vi "BottomStacking.vi"(8 "Activating Button":bool, 11 "Cancel Button":bool) -> ()   [LabVIEW 2014]
uses:
  BottomStacking.ctl
  Robot Global Data.vi
  <vilib>/Rock Robotics/WPI/RobotDrive/WPI_RobotDriveGetSetRefNum.vi
  <vilib>/Rock Robotics/WPI/RobotDrive/WPI_RobotDriveArcadeDrive_Standard(NoSaturation).vi
panel:
  in  "State Machine":T1
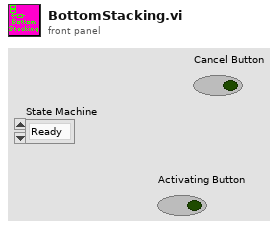
[diagram p1: front panel]
types:
  T1 = typedef "BottomStacking.ctl" = enum16{"Ready", "Raise To Stack Height", "Eject Internal Stack", "Set Down On Stack", "Release Tote", "Back Away", "Reset", "Emergency Stop"}
  T2 = typedef "WPI_SwitchDevRef.ctl" = cluster{"DevStatus":errorcluster, "DIO Channel":T3, "Controller":T4, "CntIndex":T5, "Normally Closed":bool}
  T3 = typedef "FPGA_DIOChannel.ctl" = enum8{"DIO 0", "DIO 1", "DIO 2", "DIO 3", "DIO 4", "DIO 5", "DIO 6", "DIO 7", "DIO 8", "DIO 9", "DIO MXP 0", "DIO MXP 1", "DIO MXP 2", "DIO MXP 3", "DIO MXP 4", "DIO MXP 5", "DIO MXP 6", "DIO MXP 7", "DIO MXP 8", "DIO MXP 9", "DIO MXP 10", "DIO MXP 11", "DIO MXP 12", "DIO MXP 13", "DIO MXP 14", "DIO MXP 15", "Invalid"}
  T4 = typedef "FPGA_TypedefDigitalModule.ctl" = enum16{"Controller 1"}
  T5 = typedef "FPGA_CounterCtrSystemIndex.ctl" = enum8{"Ctr 0", "Ctr 1", "Ctr 2", "Ctr 3", "Ctr 4", "Ctr 5", "Ctr 6", "Ctr 7", "Invalid"}
  T6 = typedef "WPI_MotorControlDeviceRef.ctl" = cluster{"DeviceStatus":errorcluster, "Type":T7, "PWM":cluster{"Controller":T4, "PWM Channel":T8, "DeadBand":T9}, "CAN":cluster{"Device Number":u8, "Control Mode":T10, "Semaphore":T11, "Max Vout":dbl, "TalonSRX Control Mode":T12}, "Invert":bool, "TransformRef":T13, "InvTransformRef":T13}
  T7 = typedef "WPI_MotorControlType.ctl" = enum16{"PWM", "CAN", "CANTalonSRX"}
  T8 = typedef "FPGA_DIOPWMChannel.ctl" = enum8{"PWM 0", "PWM 1", "PWM 2", "PWM 3", "PWM 4", "PWM 5", "PWM 6", "PWM 7", "PWM 8", "PWM 9", "PWM MXP 0", "PWM MXP 1", "PWM MXP 2", "PWM MXP 3", "PWM MXP 4", "PWM MXP 5", "PWM MXP 6", "PWM MXP 7", "PWM MXP 8", "PWM MXP 9", "Invalid"}
  T9 = typedef "WPI_PWMDeadband.ctl" = cluster{"Name":string, "maxPositivePwm":i32, "minPositivePwm":i32, "centerPwm":i32, "maxNegativePwm":i32, "minNegativePwm":i32, "angularRange":u16}
  T10 = typedef "WPI_CANJaguar_ControlMode.ctl" = enum8{"Percent VBus", "Current", "Speed", "Position", "Voltage"}
  T11 = typedef "Semaphore RefNum" = refnum<k1>
  T12 = typedef "WPI_CANTalonSRX_APIControlMode.ctl" = enum8{"Percent VBus", "Speed", "Position", "Slave", "Unchanged / Invalid"}
  T13 = typedef "WPI_PWMTransform_ConPane.ctl" = refnum<vi>
  T14 = typedef "WPI_RobotDriveDevRef.ctl" = cluster{"DevStatus":errorcluster, "Motors[]":T6[], "Square Inputs":bool, "Max Output":dbl}
  T15 = typedef "WPI_CANTalonSRX_GlobalStatus.ctl" = cluster{"Applied Throttle":dbl, "Module Enabled":bool, "CAN Error":errorcluster, "Closed Loop Error":dbl, "Forward Limit Switch Closed":bool, "Reverse Limit Switch Closed":bool, "Sensor Position":dbl, "Sensor Velocity":dbl, "Current":dbl, "Sticky Fault - Over Temp":bool, "Sticky Fault - Under Voltage":bool, "Sticky Fault - Forward Limit":bool, "Sticky Fault - Reverse Limit":bool, "Sticky Fault - Forward Soft Limit":bool, "Sticky Fault - Reverse Soft Limit":bool, "Brake is Enabled":bool, "Encoder Position":dbl, "Encoder Velocity":dbl, "Encoder Index Count":dbl, "Encoder A Pin State":bool, "Encoder B Pin State":bool, "Encoder Index Pin State":bool, "Analog In":dbl, "Analog In Velocity":dbl, "Temperature (C)":dbl, "Battery Voltage":dbl}
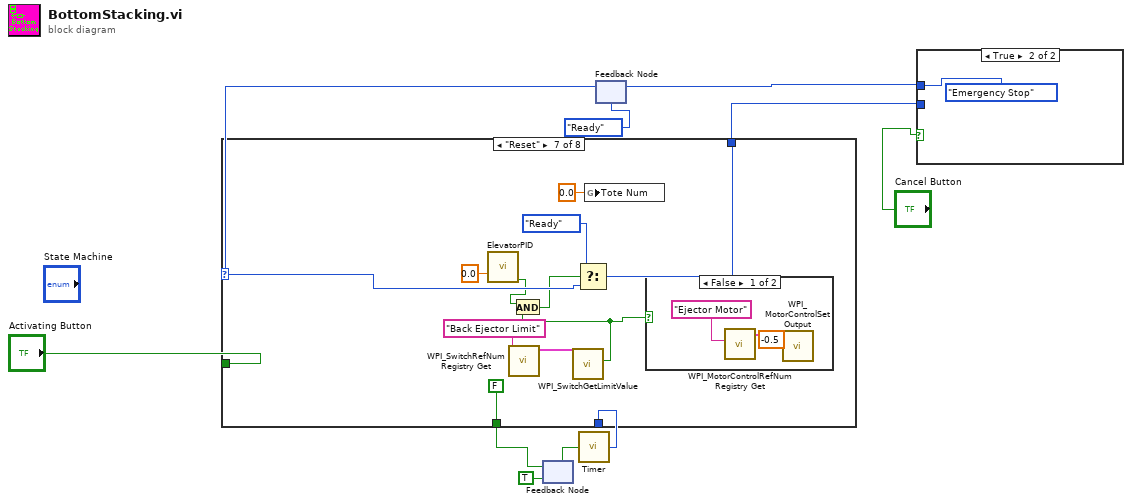
[diagram p0: block diagram]
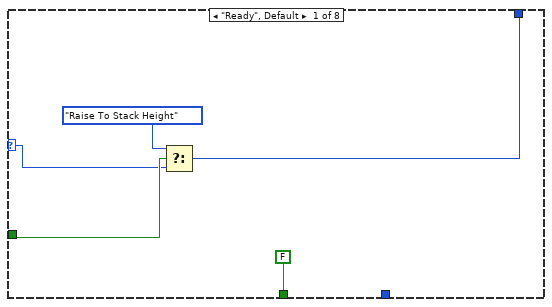
[diagram p3: hidden frame]
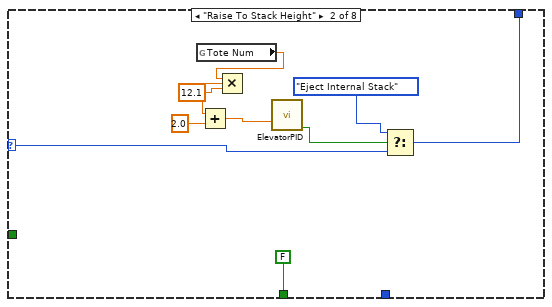
[diagram p4: hidden frame]
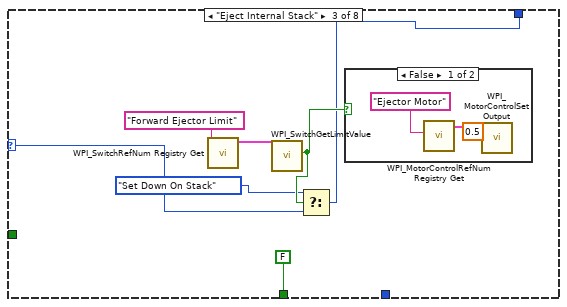
[diagram p5: hidden frame]
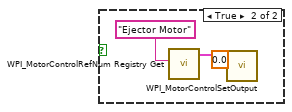
[diagram p6: hidden frame]
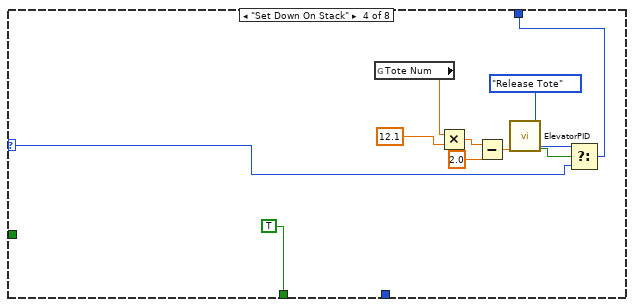
[diagram p7: hidden frame]
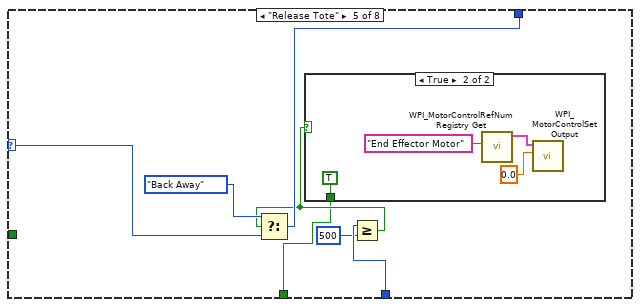
[diagram p8: hidden frame]
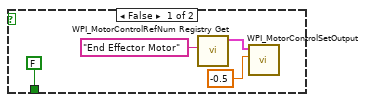
[diagram p9: hidden frame]
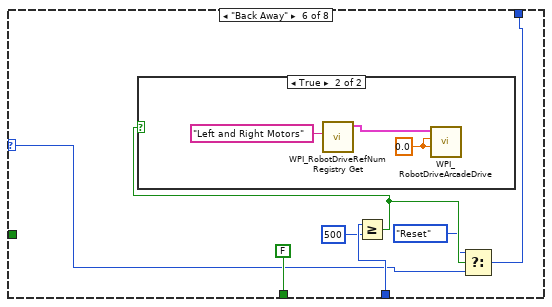
[diagram p10: hidden frame]
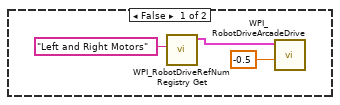
[diagram p11: hidden frame]
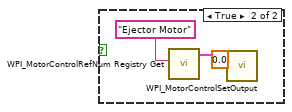
[diagram p12: hidden frame]
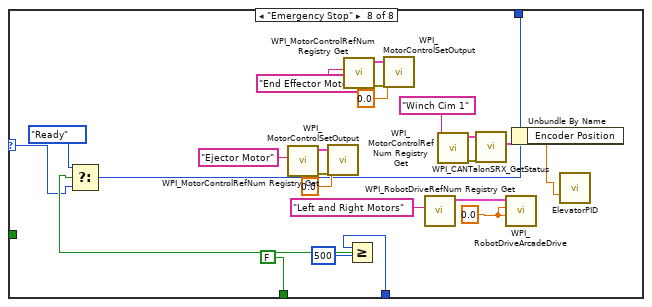
[diagram p13: hidden frame]
diagram:
  n1 = feedback #1(TRUE) -> (w7:bool)
  n2 = call "Timer.vi"("Set Timer"=w7) -> ("Time elapsed"=w5:u64)
  n3 = feedback #2(BottomStacking."Ready" ("State Machine")) -> (w9:T1)
  n4 = case shown="\"Reset\"" w9 {
    selector: w9 -> [w11 w23 w28 w42 w55 w66 w84 w97]
    tunnel: "Activating Button" -> [w15 _ _ _ _ _ _ _]
    tunnel: [w13 w22 w29 w43 w54 w64 w85 w95] -> w2
    tunnel: [FALSE FALSE FALSE TRUE w49 FALSE FALSE FALSE] -> w6
    tunnel: w5 -> [_ _ _ _ w52 w69 _ w99]
    frame "Ready", Default {
      n5 = Select(t=BottomStacking."Raise To Stack Height" ("State Machine"), s=w15, f=w11) -> (s? t:f=w13:T1)
    }
    frame "Raise To Stack Height" {
      n6 = global read "Robot Global Data.vi" "Tote Num"() -> (w19:dbl)
      n7 = Multiply(x=w19, y=12.1 ("Elevator Setpoint")) -> (x*y=w18:dbl)
      n8 = Add(x=w18, y=2.0) -> (x+y=w17:dbl)
      n9 = call "ElevatorPID.vi"("Elevator Setpoint"=w17) -> ("At Setpoint"=w24:bool)  [unwired: 14 in]
      n10 = Select(t=BottomStacking."Eject Internal Stack" ("State Machine"), s=w24, f=w23) -> (s? t:f=w22:T1)
    }
    frame "Eject Internal Stack" {
      n11 = call <vilib>:"WPI_SwitchRefNum Registry Get.vi"("refnum name"="Forward Ejector Limit") -> ("SwitchDevRef"=w31:T2)  [unwired: 9 in, 1 out]
      n12 = call <vilib>:"WPI_SwitchGetLimitValue.vi"("SwitchDevRef"=w31) -> ("Switch Pressed"=w30:bool)  [unwired: 8 in, 2 out]
      n13 = Select(t=BottomStacking."Set Down On Stack" ("State Machine"), s=w30, f=w28) -> (s? t:f=w29:T1)
      n14 = case shown="False" w30 {
        frame False {
          n15 = call <vilib>:"WPI_MotorControlRefNum Registry Get.vi"("refnum name"="Ejector Motor") -> ("MotorControlDevRef"=w35:T6)  [unwired: 9 in, 1 out]
          n16 = call <vilib>:"WPI_MotorControlSetOutput.vi"("Output"=0.5, "MotorControlDevRef"=w35) -> ()  [unwired: 7 in, 3 out]
        }
        frame True {
          n17 = call <vilib>:"WPI_MotorControlRefNum Registry Get.vi"("refnum name"="Ejector Motor") -> ("MotorControlDevRef"=w38:T6)  [unwired: 9 in, 1 out]
          n18 = call <vilib>:"WPI_MotorControlSetOutput.vi"("Output"=0.0, "MotorControlDevRef"=w38) -> ()  [unwired: 7 in, 3 out]
        }
      }
    }
    frame "Set Down On Stack" {
      n19 = global read "Robot Global Data.vi" "Tote Num"() -> (w39:dbl)
      n20 = Multiply(x=w39, y=12.1 ("Elevator Setpoint")) -> (x*y=w47:dbl)
      n21 = Subtract(x=w47, y=2.0) -> (x-y=w46:dbl)
      n22 = call "ElevatorPID.vi"("Elevator Setpoint"=w46) -> ("At Setpoint"=w44:bool)  [unwired: 14 in]
      n23 = Select(t=BottomStacking."Release Tote" ("State Machine"), s=w44, f=w42) -> (s? t:f=w43:T1)
    }
    frame "Release Tote" {
      n24 = Greater Or Equal?(x=w52, y=u64 500) -> (x >= y?=w50:bool)
      n25 = Select(t=BottomStacking."Back Away" ("State Machine"), s=w50, f=w55) -> (s? t:f=w54:T1)
      n26 = case shown="True" w50 {
        tunnel: [FALSE TRUE] -> w49
        frame False {
          n27 = call <vilib>:"WPI_MotorControlRefNum Registry Get.vi"("refnum name"="End Effector Motor") -> ("MotorControlDevRef"=w58:T6)  [unwired: 9 in, 1 out]
          n28 = call <vilib>:"WPI_MotorControlSetOutput.vi"("Output"=-0.5, "MotorControlDevRef"=w58) -> ()  [unwired: 7 in, 3 out]
        }
        frame True {
          n29 = call <vilib>:"WPI_MotorControlRefNum Registry Get.vi"("refnum name"="End Effector Motor") -> ("MotorControlDevRef"=w63:T6)  [unwired: 9 in, 1 out]
          n30 = call <vilib>:"WPI_MotorControlSetOutput.vi"("Output"=0.0, "MotorControlDevRef"=w63) -> ()  [unwired: 7 in, 3 out]
        }
      }
    }
    frame "Back Away" {
      n31 = Greater Or Equal?(x=w69, y=u64 500) -> (x >= y?=w67:bool)
      n32 = case shown="True" w67 {
        frame False {
          n33 = call <vilib>:"WPI_RobotDriveRefNum Registry Get.vi"("refnum name"="Left and Right Motors") -> ("RobotDriveDevRef"=w72:T14)  [unwired: 9 in, 1 out]
          n34 = call-poly <vilib>:"WPI_RobotDriveArcadeDrive.vi"("Y axis value"=-0.5, "RobotDriveDevRef"=w72) -> ()  [unwired: 7 in, 3 out]
        }
        frame True {
          w74 = 0.0 ("Y axis value")
          n35 = call <vilib>:"WPI_RobotDriveRefNum Registry Get.vi"("refnum name"="Left and Right Motors") -> ("RobotDriveDevRef"=w76:T14)  [unwired: 9 in, 1 out]
          n36 = call-poly <vilib>:"WPI_RobotDriveArcadeDrive.vi"("Y axis value"=w74, "X axis value"=w74, "RobotDriveDevRef"=w76) -> ()  [unwired: 6 in, 3 out]
        }
      }
      n37 = Select(t=BottomStacking."Reset" ("State Machine"), s=w67, f=w66) -> (s? t:f=w64:T1)
    }
    frame "Reset" {
      n38 = call "ElevatorPID.vi"("Elevator Setpoint"=0.0) -> ("At Setpoint"=w78:bool)  [unwired: 14 in]
      n39 = call <vilib>:"WPI_SwitchRefNum Registry Get.vi"("refnum name"="Back Ejector Limit") -> ("SwitchDevRef"=w80:T2)  [unwired: 9 in, 1 out]
      n40 = call <vilib>:"WPI_SwitchGetLimitValue.vi"("SwitchDevRef"=w80) -> ("Switch Pressed"=w79:bool)  [unwired: 8 in, 2 out]
      n41 = And(x=w78, y=w79) -> (x .and. y?=w82:bool)
      n42 = Select(t=BottomStacking."Ready" ("State Machine"), s=w82, f=w84) -> (s? t:f=w85:T1)
      n43 = global write "Robot Global Data.vi" "Tote Num"(0.0 ("Tote Num")) -> ()
      n44 = case shown="False" w79 {
        frame False {
          n45 = call <vilib>:"WPI_MotorControlRefNum Registry Get.vi"("refnum name"="Ejector Motor") -> ("MotorControlDevRef"=w90:T6)  [unwired: 9 in, 1 out]
          n46 = call <vilib>:"WPI_MotorControlSetOutput.vi"("Output"=-0.5, "MotorControlDevRef"=w90) -> ()  [unwired: 7 in, 3 out]
        }
        frame True {
          n47 = call <vilib>:"WPI_MotorControlRefNum Registry Get.vi"("refnum name"="Ejector Motor") -> ("MotorControlDevRef"=w93:T6)  [unwired: 9 in, 1 out]
          n48 = call <vilib>:"WPI_MotorControlSetOutput.vi"("Output"=0.0, "MotorControlDevRef"=w93) -> ()  [unwired: 7 in, 3 out]
        }
      }
    }
    frame "Emergency Stop" {
      w108 = 0.0 ("Output")
      n49 = call <vilib>:"WPI_MotorControlRefNum Registry Get.vi"("refnum name"="Ejector Motor") -> ("error out"=w109:errorcluster, "MotorControlDevRef"=w110:T6)  [unwired: 9 in]
      n50 = call <vilib>:"WPI_MotorControlSetOutput.vi"("error in (no error)"=w109, "Output"=0.0, "MotorControlDevRef"=w110) -> ()  [unwired: 6 in, 3 out]
      n51 = call <vilib>:"WPI_MotorControlRefNum Registry Get.vi"("refnum name"="End Effector Motor") -> ("error out"=w113:errorcluster, "MotorControlDevRef"=w114:T6)  [unwired: 9 in]
      n52 = Greater Or Equal?(x=w99, y=u64 500) -> (x >= y?=w98:bool)
      n53 = Select(t=BottomStacking."Ready" ("State Machine"), s=w98, f=w97) -> (s? t:f=w95:T1)
      n54 = call <vilib>:"WPI_MotorControlSetOutput.vi"("error in (no error)"=w113, "Output"=0.0, "MotorControlDevRef"=w114) -> ()  [unwired: 6 in, 3 out]
      n55 = call <vilib>:"WPI_RobotDriveRefNum Registry Get.vi"("refnum name"="Left and Right Motors") -> ("RobotDriveDevRef"=w107:T14)  [unwired: 9 in, 1 out]
      n56 = call <vilib>:"WPI_MotorControlRefNum Registry Get.vi"("refnum name"="Winch Cim 1") -> ("error out"=w105:errorcluster, "MotorControlDevRef"=w104:T6)  [unwired: 9 in]
      n57 = call <vilib>:"WPI_CANTalonSRX_GetStatus.vi"("error in (no error)"=w105, "CAN Talon SRX Ref"=w104) -> ("Talon SRX Status"=w102:T15)  [unwired: 7 in, 2 out]
      n58 = call-poly <vilib>:"WPI_RobotDriveArcadeDrive.vi"("Y axis value"=w108, "X axis value"=w108, "RobotDriveDevRef"=w107) -> ()  [unwired: 6 in, 3 out]
      n59 = Unbundle By Name(w102) -> ("Encoder Position"=w94:dbl)
      n60 = call "ElevatorPID.vi"("Elevator Setpoint"=w94) -> ()  [unwired: 14 in, 1 out]
    }
  }
  n61 = feedback-in #1(w6) -> ()
  n62 = case shown="True" "Cancel Button" {
    tunnel: [w117 BottomStacking."Emergency Stop" ("State Machine")] -> w3
    tunnel: w2 -> [w117 _]
    frame False {
    }
    frame True {
    }
  }
  n63 = feedback-in #2(w3) -> ()
